vi "exnSpectralBlock spectral measurements RMS poly.vi"   [LabVIEW 2017]
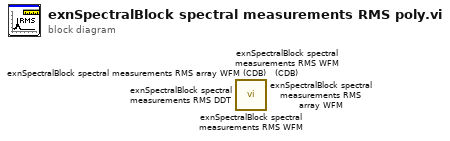
[diagram p0: block diagram]
diagram:
  n1 = call <vilib>:"exnSpectralBlock spectral measurements RMS WFM.vi"() -> ()  [unwired: 12 in, 4 out]
  n2 = call <vilib>:"exnSpectralBlock spectral measurements RMS WFM (CDB).vi"() -> ()  [unwired: 12 in, 4 out]
  n3 = call <vilib>:"exnSpectralBlock spectral measurements RMS DDT.vi"() -> ()  [unwired: 12 in, 4 out]
  n4 = call <vilib>:"exnSpectralBlock spectral measurements RMS array WFM.vi"() -> ()  [unwired: 12 in, 4 out]
  n5 = call <vilib>:"exnSpectralBlock spectral measurements RMS array WFM (CDB).vi"() -> ()  [unwired: 12 in, 4 out]
